vi "State_Machine.vi"() -> ()   [LabVIEW 2020]
uses:
  Enum_Type_Def.ctl
panel:
  in  "Milliseconds to wait":u32=1000
  out "While Cycle Nr.":i32
  in  "Start":bool
  out "State Machine Status":string
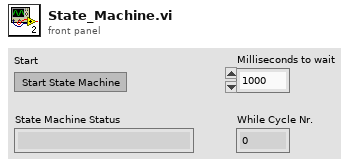
[diagram p1: front panel]
types:
  T1 = typedef "Enum_Type_Def.ctl" = enum16{"Waiting for Event", "Initialization", "Calculation", "Representation"}
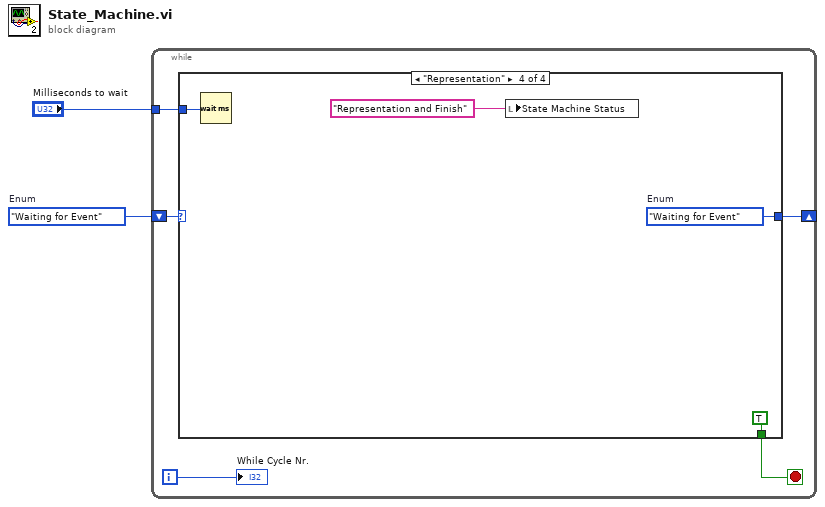
[diagram p0: block diagram]
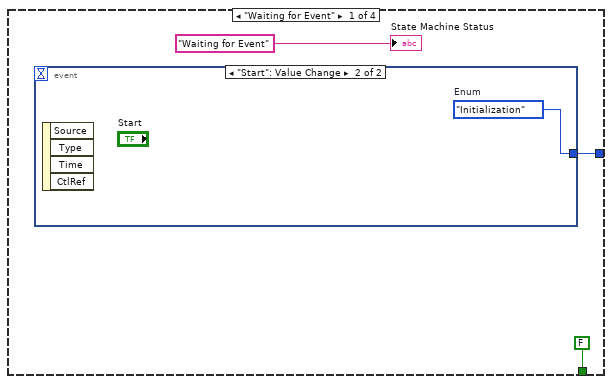
[diagram p2: hidden frame]
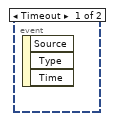
[diagram p3: hidden frame]
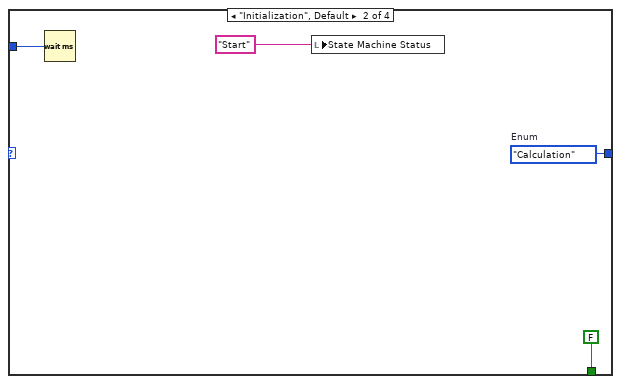
[diagram p4: hidden frame]
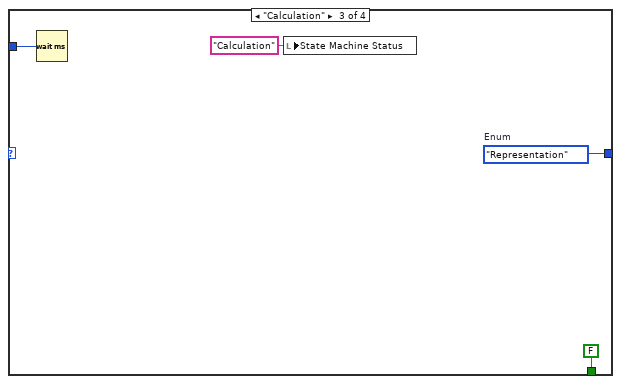
[diagram p5: hidden frame]
diagram:
  w2 = Enum_Type_Def."Waiting for Event"  # Enum
  n1 = while {
    shift-right: [w6] -> _
    shift-left: w2 -> [w7]
    tunnel: "Milliseconds to wait" -> [w3]
    i -> [w4]
    stop <- w5 stop-if-true
    n2 = case shown="\"Representation\"" w7 {
      tunnel: [w10 w15 w19 w21] -> w6
      tunnel: [FALSE FALSE FALSE TRUE] -> w5
      tunnel: w3 -> [_ w12 w16 w20]
      frame "Waiting for Event" {
        n3 = event shown="[1] \"Start\": Value Change" {
          selector: _ -> [_ _]
          dyn-events: _ -> [_ _]
          timeout: _ -> [_ _]
          tunnel: [_ w11] -> w10
          event Timeout {
            n4 = event-data() -> ()  [unwired: 1 in, 3 out]
          }
          event "Start": Value Change {
            w11 = Enum_Type_Def."Initialization"  # Enum
            n5 = event-data() -> ()  [unwired: 1 in, 4 out]
          }
        }
        "State Machine Status" <- "Waiting for Event" ("State Machine Status")
      }
      frame "Initialization", Default {
        w15 = Enum_Type_Def."Calculation"  # Enum
        n6 = Wait (ms)(milliseconds to wait=w12) -> ()  [unwired: 1 out]
        n7 = local write "State Machine Status"("Start") -> ()
      }
      frame "Calculation" {
        w19 = Enum_Type_Def."Representation"  # Enum
        n8 = Wait (ms)(milliseconds to wait=w16) -> ()  [unwired: 1 out]
        n9 = local write "State Machine Status"("Calculation" ("String 2")) -> ()
      }
      frame "Representation" {
        w21 = Enum_Type_Def."Waiting for Event"  # Enum
        n10 = Wait (ms)(milliseconds to wait=w20) -> ()  [unwired: 1 out]
        n11 = local write "State Machine Status"("Representation and Finish" ("String")) -> ()
      }
    }
    "While Cycle Nr." <- w4
  }
